vi "XY date manual remove data pts.vi"() -> ()   [LabVIEW 2021]
panel:
  in  "Undo":bool
  out "y-array out":dbl[](array[numeric])
  out "x-array out":dbl[](array[numeric])
  out "removed pts index":i32[](array[numeric])
  in  "method":T1(ring)
  in  "OK Button":bool
  out "zoom scale":T2
  in  "stop":bool
  in  "y-array":dbl[](array[numeric])
  in  "x-array":dbl[](array[numeric])
  out "XY Graph":cluster{"x-array":dbl[], "y-array":dbl[]}(graph)
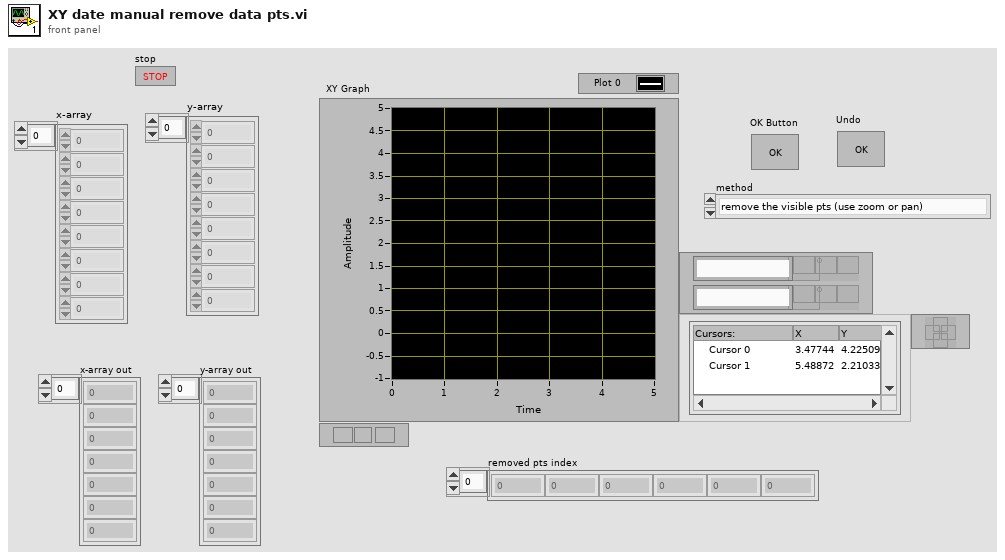
[diagram p1: front panel]
types:
  T1 = enum16{"remove the visible pts (use zoom or pan)", "remove pts inside rectangle defined by cursors"}
  T2 = cluster{"XScale.Minimum":dbl, "XScale.Maximum":dbl, "YScale.Minimum":dbl, "YScale.Maximum":dbl}
  T3 = typedef "LVCursorListTypeDef.ctl" = cluster{"Name":string, "Color":u32, "Style":u8, "Point Style":u8, "Name Visible":bool, "Allow Drag":bool, "Cursor Mode":u32, "Plot":i32, "Index":i32, "Position":cluster{"X":dbl, "Y":dbl}, "X Scale":u32, "Y Scale":u32, "Watch Plots":i32[], "Watch All Plots":bool, "Plot Area":i32, "Label Offset":cluster{"X":dbl, "Y":dbl}}[]
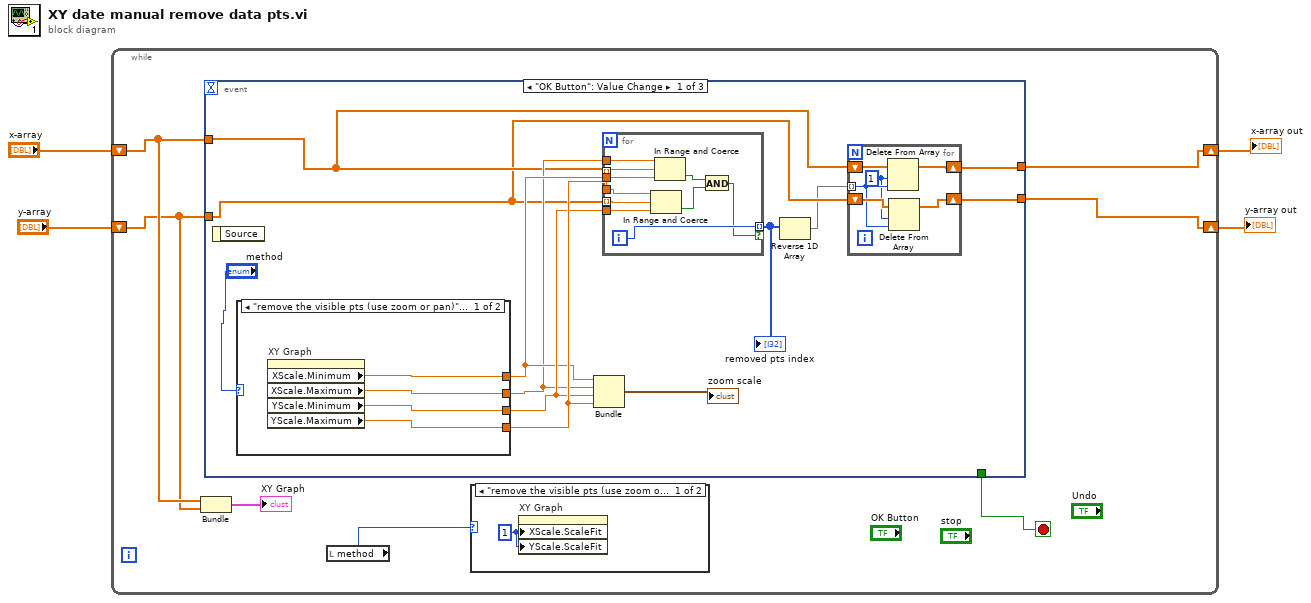
[diagram p0: block diagram]
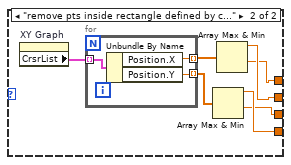
[diagram p3: hidden frame]
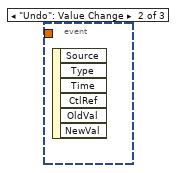
[diagram p4: hidden frame]
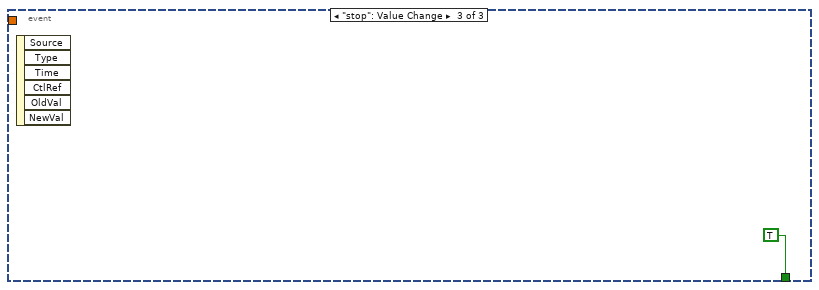
[diagram p5: hidden frame]
diagram:
  n1 = while {
    shift-right: [w8] -> w2
    shift-left: "x-array" -> [w11]
    shift-right: [w7] -> w1
    shift-left: "y-array" -> [w10]
    stop <- w5 stop-if-true
    n2 = Bundle("x-array"=w11, "y-array"=w10) -> (→"XY Graph":cluster{"x-array":dbl[], "y-array":dbl[]})  [unwired: 1 in]
    n3 = event shown="[0] \"OK Button\": Value Change" {
      selector: _ -> [_ _ _]
      dyn-events: _ -> [_ _ _]
      timeout: _ -> [_ _ _]
      tunnel: w11 -> [w18 _ _]
      tunnel: w10 -> [w17 _ _]
      tunnel: [w15 _ _] -> w8
      tunnel: [w14 _ _] -> w7
      tunnel: [_ _ TRUE] -> w5
      event "OK Button": Value Change {
        n4 = event-data() -> ()  [unwired: 1 in, 1 out]
        n5 = case shown="\"remove the visible pts (use zoom or pan)\", Default" "method" {
          tunnel: [w28 w30] -> w24
          tunnel: [w27 w29] -> w23
          tunnel: [w26 w31] -> w22
          tunnel: [w25 w32] -> w21
          frame "remove the visible pts (use zoom or pan)", Default {
            n6 = property on="XY Graph" class="XYGraph (strict)"() -> ("XScale.Minimum"=w26:dbl, "XScale.Maximum"=w25:dbl, "YScale.Minimum"=w27:dbl, "YScale.Maximum"=w28:dbl)  [unwired: 2 in, 2 out]
          }
          frame "remove pts inside rectangle defined by cursors" {
            n7 = property on="XY Graph" class="XYGraph (strict)"() -> ("CrsrList"=w35:T3)  [unwired: 2 in, 2 out]
            n8 = for {
              tunnel: w35 -> [w38] mode=indexing
              tunnel: [w37] -> w34 mode=indexing
              tunnel: [w36] -> w33 mode=indexing
              n9 = Unbundle By Name(w38) -> ("Position.X"=w37:dbl, "Position.Y"=w36:dbl)
            }
            n10 = Array Max & Min(array=w33) -> (max value=w30:dbl, min value=w29:dbl)  [unwired: 2 out]
            n11 = Array Max & Min(array=w34) -> (max value=w32:dbl, min value=w31:dbl)  [unwired: 2 out]
          }
        }
        n12 = Bundle("XScale.Minimum"=w22, "XScale.Maximum"=w21, "YScale.Minimum"=w23, "YScale.Maximum"=w24) -> (→"zoom scale":T2)  [unwired: 1 in]
        n13 = for {
          tunnel: w18 -> [w54] mode=indexing
          tunnel: w17 -> [w49] mode=indexing
          tunnel: w24 -> [w48]
          tunnel: [w51] -> w19 mode=indexing if=w50
          tunnel: w23 -> [w47]
          tunnel: w21 -> [w46]
          tunnel: w22 -> [w45]
          i -> [w51]
          n14 = In Range and Coerce(upper limit=w48, x=w49, lower limit=w47) -> (In Range?=w53:bool)  [unwired: 1 out]
          n15 = In Range and Coerce(upper limit=w46, x=w54, lower limit=w45) -> (In Range?=w52:bool)  [unwired: 1 out]
          n16 = And(x=w52, y=w53) -> (x .and. y?=w50:bool)
        }
        "removed pts index" <- w19
        n17 = Reverse 1D Array(array=w19) -> (reversed array=w16:i32[])
        n18 = for {
          tunnel: w16 -> [w40] mode=indexing
          shift-right: [w42] -> w15
          shift-left: w18 -> [w44]
          shift-right: [w41] -> w14
          shift-left: w17 -> [w43]
          w39 = 1 ("length")
          n19 = Delete From Array(array=w44, length=w39, index=w40) -> (array with subset deleted=w42:dbl[])  [unwired: 1 out]
          n20 = Delete From Array(array=w43, length=w39, index=w40) -> (array with subset deleted=w41:dbl[])  [unwired: 1 out]
        }
      }
      event "Undo": Value Change {
        n21 = event-data() -> ()  [unwired: 1 in, 6 out]
      }
      event "stop": Value Change {
        n22 = event-data() -> ()  [unwired: 1 in, 6 out]
      }
    }
    n23 = local read "method"() -> (w6:T1)
    n24 = case shown="\"remove the visible pts (use zoom or pan)\", Default" w6 {
      frame "remove the visible pts (use zoom or pan)", Default {
        w12 = u8 1 ("X Scale.Scale Fit")
        n25 = property on="XY Graph" class="XYGraph (strict)"("XScale.ScaleFit"=w12, "YScale.ScaleFit"=w12) -> ()  [unwired: 2 in, 2 out]
      }
      frame "remove pts inside rectangle defined by cursors" {
      }
    }
  }
  "y-array out" <- w1
  "x-array out" <- w2
